vi "3D Quadrature (VI).vi"(7 "data":variant, 8 "tolerance":dbl=1e-05, 9 "Lower Limits":T1, 10 "Upper Limits":T2={"x upper limit"=1.0, "y upper limit"=1.0, "z upper limit"=1.0}, 11 "integrand":refnum<vi>) -> (0 "error":i32, 3 "result":dbl)   [LabVIEW 2020, in "NI_AALPro.lvlib"]
doc: "Performs numerical integration using adaptive quadrature approach. You must manually select the polymorphic instance to use."
uses:
  <vilib>/Analysis/NI_AALPro.lvlib
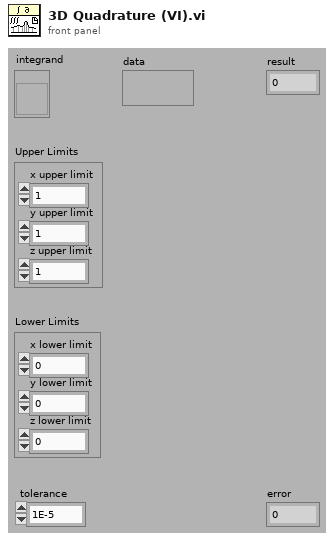
[diagram p1: front panel]
types:
  T1 = cluster{"x lower limit":dbl, "y lower limit":dbl, "z lower limit":dbl}
  T2 = cluster{"x upper limit":dbl, "y upper limit":dbl, "z upper limit":dbl}
  T3 = cluster{"x lower limit":dbl, "x upper limit":dbl}
  T4 = cluster{"y lower limit":dbl, "y upper limit":dbl}
  T5 = cluster{"z lower limit":dbl, "z upper limit":dbl}
  T6 = cluster{cluster{"x lower limit":dbl, "x upper limit":dbl}, cluster{"y lower limit":dbl, "y upper limit":dbl}, cluster{"z lower limit":dbl, "z upper limit":dbl}}
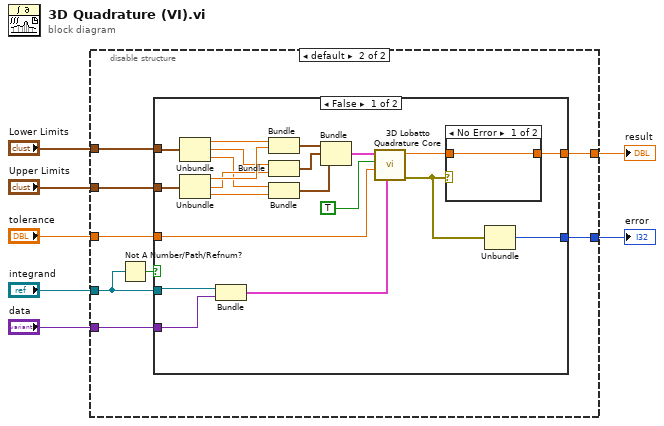
[diagram p0: block diagram]
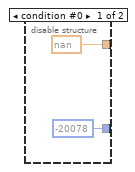
[diagram p2: hidden frame]
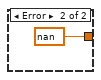
[diagram p3: hidden frame]
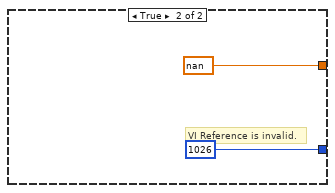
[diagram p4: hidden frame]
diagram:
  n1 = disable-structure shown="default" {
    disable-tunnel: [-20078 ("code") w17] -> w7
    disable-tunnel: "tolerance" -> [_ w16]
    disable-tunnel: [nan ("result") w15] -> w5
    disable-tunnel: "integrand" -> [_ w13]
    disable-tunnel: "data" -> [_ w12]
    disable-tunnel: "Lower Limits" -> [_ w11]
    disable-tunnel: "Upper Limits" -> [_ w10]
    frame condition #0 {
    }
    frame condition #1 (active) {
      n2 = Not A Number/Path/Refnum?(number/path/refnum=w13) -> (NaN/Path/Refnum?=w14:bool)
      n3 = case shown="False" w14 {
        tunnel: [w38 nan] -> w15
        tunnel: [w37 1026] -> w17
        tunnel: w16 -> [w36 _]
        tunnel: w13 -> [w21 _]
        tunnel: w12 -> [w20 _]
        tunnel: w11 -> [w33 _]
        tunnel: w10 -> [w32 _]
        frame False {
          n4 = Unbundle(w33) -> ("x lower limit"=w31:dbl, "y lower limit"=w29:dbl, "z lower limit"=w27:dbl)
          n5 = Unbundle(w32) -> ("x upper limit"=w30:dbl, "y upper limit"=w28:dbl, "z upper limit"=w26:dbl)
          n6 = Bundle("integrand"=w21, "data"=w20) -> (w19:cluster{"integrand":refnum<vi>, "data":variant})  [unwired: 1 out]
          n7 = Bundle("x lower limit"=w31, "x upper limit"=w30) -> (w24:T3)  [unwired: 1 out]
          n8 = Bundle("y lower limit"=w29, "y upper limit"=w28) -> (w23:T4)  [unwired: 1 out]
          n9 = Bundle("z lower limit"=w27, "z upper limit"=w26) -> (w22:T5)  [unwired: 1 out]
          n10 = Bundle(w24, w23, w22) -> (w25:T6)  [unwired: 1 out]
          n11 = call <vilib>:"3D Lobatto Quadrature Core.vi"("VI ref"=w19, "tolerance"=w36, "Formula/VI ref"=TRUE, "limits"=w25) -> ("error out"=w34:errorcluster, "result"=w35:dbl)  [unwired: 1 in, 5 out]
          n12 = case shown="No Error" w34 {
            tunnel: w35 -> [w39 _]
            tunnel: [w39 nan] -> w38
            frame No Error {
            }
            frame Error {
            }
          }
          n13 = Unbundle(w34) -> ("code"=w37:i32)  [unwired: 2 out]
        }
        frame True {
          # "VI Reference is invalid."
        }
      }
    }
  }
  "error" <- w7
  "result" <- w5
